vi "Manager Initialize.vi"(8 "error in":errorcluster) -> (0 "error out":errorcluster)   [LabVIEW 2020, in "Manager.lvlib"]
uses:
  Manager.lvlib
  Eventing/Event FGV Actions.ctl
panel:
  # "Event Handler: Initialize"
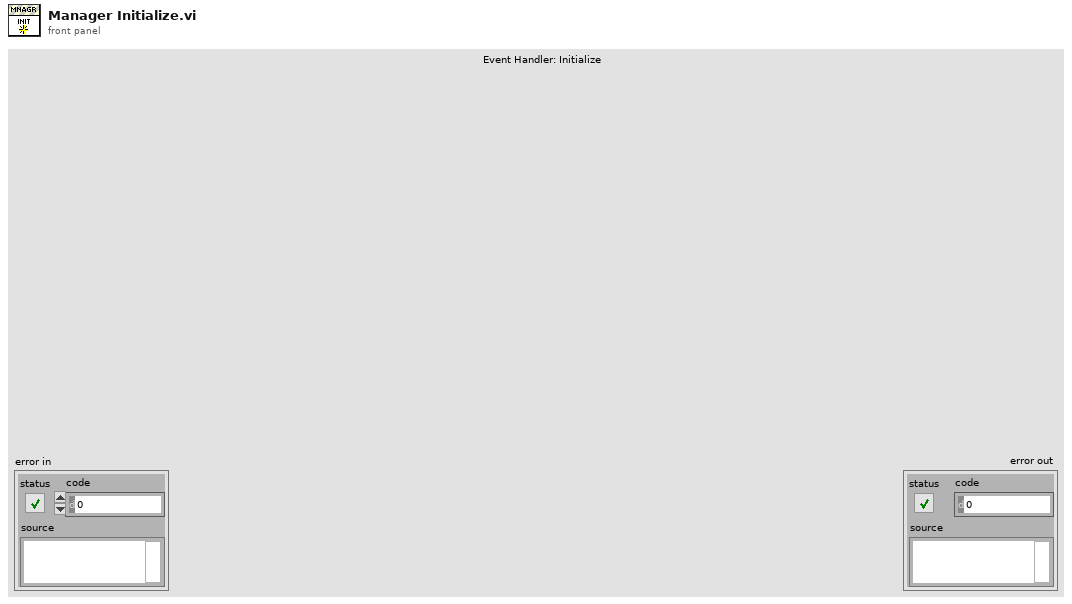
[diagram p1: front panel]
types:
  T1 = typedef "Manager.lvlib/Event FGV Actions.ctl" = enum16{"Get", "Create", "Destroy"}
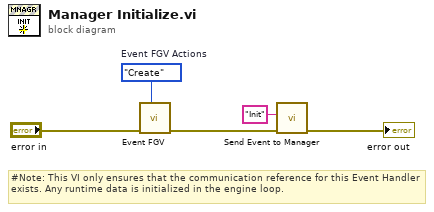
[diagram p0: block diagram]
diagram:
  w5 = Event_FGV_Actions."Create"  # Event FGV Actions
  # "#Note: This VI only ensures that the communication reference for this Event Handler exists. Any runtime data is initialized in the engine loop."
  n1 = call "Event FGV.vi"("Event FGV Actions"=w5, "error in"="error in") -> ("error out"=w2:errorcluster)  [unwired: 7 in, 2 out]
  n2 = call "Send Event to Manager.vi"("error in"=w2, "Command"="Init") -> ("error out"=→"error out":errorcluster)  [unwired: 9 in]
